vi "Weather Parse Test.vi"() -> ()   [LabVIEW 2020, in "CDM-Config.lvlib"] (continued)
    \"UGC\": [\n                        \"PKZ662\"\n                    ]\n                },\n                \"affectedZones\": [\n                    \"https://api.weather.gov/zones/forecast/PKZ662\"\n                ],\n                \"references\": [],\n                \"sent\": \"2025-12-02T14:58:00-09:00\",\n                \"effective\": \"2025-12-02T14:58:00-09:00\",\n                \"onset\": \"2025-12-02T14:00:00-09:00\",\n                \"expires\": \"2025-12-03T09:00:00-09:00\",\n                \"ends\": \"2025-12-03T17:00:00-09:00\",\n                \"status\": \"Actual\",\n                \"messageType\": \"Alert\",\n                \"category\": \"Met\",\n                \"severity\": \"Minor\",\n                \"certainty\": \"Likely\",\n                \"urgency\": \"Expected\",\n                \"event\": \"Small Craft Advisory\",\n                \"sender\": \"w-nws.webmaster@noaa.gov\",\n                \"senderName\": \"NWS Juneau AK\",\n                \"headline\": \"Small Craft Advisory issued December 2 at 2:58PM AKST until December 3 at 5:00PM AKST by NWS Juneau AK\",\n                \"description\": \"Southeast Alaska Coastal Waters from Dixon Entrance to\\nCape Suckling out 100 NM\\n\\nWind forecasts reflect the predominant speed and direction\\nexpected. Seas forecasts represent the average of the highest\\none-third of the combined windwave and swell height.\\n\\n.TONIGHT...S wind 25 kt. Seas 11 ft. Rain.\\n.WED...SW wind 15 kt. Seas 11 ft. SW swell.\\n.WED NIGHT...W wind 20 kt. Seas 10 ft.\\n.THU...W wind 10 kt. Seas 9 ft.\\n.THU NIGHT...SE wind 20 kt. Seas 9 ft.\\n.FRI...W wind 25 kt. Seas 14 ft.\\n.SAT...S wind 30 kt. Seas 17 ft.\\n.SUN...SW gale to 35 kt. Seas 20 ft.\",\n                \"instruction\": null,\n                \"response\": \"Avoid\",\n                \"parameters\": {\n                    \"AWIPSidentifier\": [\n                        \"CWFAEG\"\n                    ],\n                    \"WMOidentifier\": [\n                        \"FZAK52 PAJK 022358\"\n                    ],\n                    \"NWSheadline\": [\n                        \"SMALL CRAFT ADVISORY THROUGH WEDNESDAY\"\n                    ],\n                    \"BLOCKCHANNEL\": [\n                        \"EAS\",\n                        \"NWEM\",\n                        \"CMAS\"\n                    ],\n                    \"VTEC\": [\n                        \"/O.NEW.PAJK.SC.Y.1226.251202T2300Z-251204T0200Z/\"\n                    ],\n                    \"eventEndingTime\": [\n                        \"2025-12-03T17:00:00-09:00\"\n                    ]\n                },\n                \"scope\": \"Public\",\n                \"code\": \"IPAWSv1.0\",\n                \"language\": \"en-US\",\n                \"web\": \"http://www.weather.gov\",\n                \"eventCode\": {\n                    \"SAME\": [\n                        \"NWS\"\n                    ],\n                    \"NationalWeatherService\": [\n                        \"SCY\"\n                    ]\n                }\n            }\n        },\n        {\n            \"id\": \"https://api.weather.gov/alerts/urn:oid:2.49.0.1.840.0.63d5e98d8e0beb997c67cb867ab3ed73fdae0812.009.1\",\n            \"type\": \"Feature\",\n            \"geometry\": null,\n            \"properties\": {\n                \"@id\": \"https://api.weather.gov/alerts/urn:oid:2.49.0.1.840.0.63d5e98d8e0beb997c67cb867ab3ed73fdae0812.009.1\",\n                \"@type\": \"wx:Alert\",\n                \"id\": \"urn:oid:2.49.0.1.840.0.63d5e98d8e0beb997c67cb867ab3ed73fdae0812.009.1\",\n                \"areaDesc\": \"Cape Spencer to Cape Fairweather from 15 to 85 NM\",\n                \"geocode\": {\n                    \"SAME\": [\n                        \"058664\"\n                    ],\n                    \"UGC\": [\n                        \"PKZ664\"\n                    ]\n                },\n                \"affectedZones\": [\n                    \"https://api.weather.gov/zones/forecast/PKZ664\"\n                ],\n                \"references\": [],\n                \"sent\": \"2025-12-02T14:58:00-09:00\",\n                \"effective\": \"2025-12-02T14:58:00-09:00\",\n                \"onset\": \"2025-12-02T14:00:00-09:00\",\n                \"expires\": \"2025-12-03T09:00:00-09:00\",\n                \"ends\": \"2025-12-03T17:00:00-09:00\",\n                \"status\": \"Actual\",\n                \"messageType\": \"Alert\",\n                \"category\": \"Met\",\n                \"severity\": \"Minor\",\n                \"certainty\": \"Likely\",\n                \"urgency\": \"Expected\",\n                \"event\": \"Small Craft Advisory\",\n                \"sender\": \"w-nws.webmaster@noaa.gov\",\n                \"senderName\": \"NWS Juneau AK\",\n                \"headline\": \"Small Craft Advisory issued December 2 at 2:58PM AKST until December 3 at 5:00PM AKST by NWS Juneau AK\",\n                \"description\": \"Southeast Alaska Coastal Waters from Dixon Entrance to\\nCape Suckling out 100 NM\\n\\nWind forecasts reflect the predominant speed and direction\\nexpected. Seas forecasts represent the average of the highest\\none-third of the combined windwave and swell height.\\n\\n.TONIGHT...SE wind 20 kt. Seas 11 ft. Rain in the evening.\\n.WED...S wind 20 kt becoming W in the afternoon. Seas\\n12 ft. SW swell.\\n.WED NIGHT...W wind 20 kt. Seas 10 ft.\\n.THU...W wind 15 kt. Seas 9 ft.\\n.THU NIGHT...SE wind 20 kt. Seas 8 ft.\\n.FRI...SW wind 25 kt. Seas 9 ft.\\n.SAT...S gale to 35 kt. Seas 14 ft.\\n.SUN...S gale to 35 kt. Seas 18 ft.\",\n                \"instruction\": null,\n                \"response\": \"Avoid\",\n                \"parameters\": {\n                    \"AWIPSidentifier\": [\n                        \"CWFAEG\"\n                    ],\n                    \"WMOidentifier\": [\n                        \"FZAK52 PAJK 022358\"\n                    ],\n                    \"NWSheadline\": [\n                        \"SMALL CRAFT ADVISORY THROUGH WEDNESDAY\"\n                    ],\n                    \"BLOCKCHANNEL\": [\n                        \"EAS\",\n                        \"NWEM\",\n                        \"CMAS\"\n                    ],\n                    \"VTEC\": [\n                        \"/O.NEW.PAJK.SC.Y.1230.251202T2300Z-251204T0200Z/\"\n                    ],\n                    \"eventEndingTime\": [\n                        \"2025-12-03T17:00:00-09:00\"\n                    ]\n                },\n                \"scope\": \"Public\",\n                \"code\": \"IPAWSv1.0\",\n                \"language\": \"en-US\",\n                \"web\": \"http://www.weather.gov\",\n                \"eventCode\": {\n                    \"SAME\": [\n                        \"NWS\"\n                    ],\n                    \"NationalWeatherService\": [\n                        \"SCY\"\n                    ]\n                }\n            }\n        },\n        {\n            \"id\": \"https://api.weather.gov/alerts/urn:oid:2.49.0.1.840.0.63d5e98d8e0beb997c67cb867ab3ed73fdae0812.013.1\",\n            \"type\": \"Feature\",\n            \"geometry\": null,\n            \"properties\": {\n                \"@id\": \"https://api.weather.gov/alerts/urn:oid:2.49.0.1.840.0.63d5e98d8e0beb997c67cb867ab3ed73fdae0812.013.1\",\n                \"@type\": \"wx:Alert\",\n                \"id\": \"urn:oid:2.49.0.1.840.0.63d5e98d8e0beb997c67cb867ab3ed73fdae0812.013.1\",\n                \"areaDesc\": \"Icy Cape to Cape Suckling from 15 to 80 NM\",\n                \"geocode\": {\n                    \"SAME\": [\n                        \"058672\"\n                    ],\n                    \"UGC\": [\n                        \"PKZ672\"\n                    ]\n                },\n                \"affectedZones\": [\n                    \"https://api.weather.gov/zones/forecast/PKZ672\"\n                ],\n                \"references\": [],\n                \"sent\": \"2025-12-02T14:58:00-09:00\",\n                \"effective\": \"2025-12-02T14:58:00-09:00\",\n                \"onset\": \"2025-12-02T14:00:00-09:00\",\n                \"expires\": \"2025-12-03T09:00:00-09:00\",\n                \"ends\": \"2025-12-03T17:00:00-09:00\",\n                \"status\": \"Actual\",\n                \"messageType\": \"Alert\",\n                \"category\": \"Met\",\n                \"severity\": \"Minor\",\n                \"certainty\": \"Likely\",\n                \"urgency\": \"Expected\",\n                \"event\": \"Small Craft Advisory\",\n                \"sender\": \"w-nws.webmaster@noaa.gov\",\n                \"senderName\": \"NWS Juneau AK\",\n                \"headline\": \"Small Craft Advisory issued December 2 at 2:58PM AKST until December 3 at 5:00PM AKST by NWS Juneau AK\",\n                \"description\": \"Southeast Alaska Coastal Waters from Dixon Entrance to\\nCape Suckling out 100 NM\\n\\nWind forecasts reflect the predominant speed and direction\\nexpected. Seas forecasts represent the average of the highest\\none-third of the combined windwave and swell height.\\n\\n.TONIGHT...E wind 25 kt. Seas 12 ft. Rain early in the evening.\\n.WED...E wind 20 kt becoming W in the afternoon. Seas\\n12 ft.\\n.WED NIGHT...W wind 15 kt. Seas 10 ft.\\n.THU...SW wind 10 kt. Seas 8 ft. SW swell.\\n.THU NIGHT...E wind 10 kt. Seas 8 ft.\\n.FRI...S wind 20 kt. Seas 8 ft.\\n.SAT...SE wind 30 kt. Seas 13 ft.\\n.SUN...SE gale to 35 kt. Seas 15 ft.\",\n                \"instruction\": null,\n                \"response\": \"Avoid\",\n                \"parameters\": {\n                    \"AWIPSidentifier\": [\n                        \"CWFAEG\"\n                    ],\n                    \"WMOidentifier\": [\n                        \"FZAK52 PAJK 022358\"\n                    ],\n                    \"NWSheadline\": [\n                        \"SMALL CRAFT ADVISORY THROUGH WEDNESDAY\"\n                    ],\n                    \"BLOCKCHANNEL\": [\n                        \"EAS\",\n                        \"NWEM\",\n                        \"CMAS\"\n                    ],\n                    \"VTEC\": [\n                        \"/O.NEW.PAJK.SC.Y.1234.251202T2300Z-251204T0200Z/\"\n                    ],\n                    \"eventEndingTime\": [\n                        \"2025-12-03T17:00:00-09:00\"\n                    ]\n                },\n                \"scope\": \"Public\",\n                \"code\": \"IPAWSv1.0\",\n                \"language\": \"en-US\",\n                \"web\": \"http://www.weather.gov\",\n                \"eventCode\": {\n                    \"SAME\": [\n                        \"NWS\"\n                    ],\n                    \"NationalWeatherService\": [\n                        \"SCY\"\n                    ]\n                }\n            }\n        },\n        {\n            \"id\": \"https://api.weather.gov/alerts/urn:oid:2.49.0.1.840.0.63d5e98d8e0beb997c67cb867ab3ed73fdae0812.002.1\",\n            \"type\": \"Feature\",\n            \"geometry\": null,\n            \"properties\": {\n                \"@id\": \"https://api.weather.gov/alerts/urn:oid:2.49.0.1.840.0.63d5e98d8e0beb997c67cb867ab3ed73fdae0812.002.1\",\n                \"@type\": \"wx:Alert\",\n                \"id\": \"urn:oid:2.49.0.1.840.0.63d5e98d8e0beb997c67cb867ab3ed73fdae0812.002.1\",\n                \"areaDesc\": \"Dixon Entrance to Cape Decision out to 15 NM\",\n                \"geocode\": {\n                    \"SAME\": [\n                        \"058641\"\n                    ],\n                    \"UGC\": [\n                        \"PKZ641\"\n                    ]\n                },\n                \"affectedZones\": [\n                    \"https://api.weather.gov/zones/forecast/PKZ641\"\n                ],\n                \"references\": [],\n                \"sent\": \"2025-12-02T14:58:00-09:00\",\n                \"effective\": \"2025-12-02T14:58:00-09:00\",\n                \"onset\": \"2025-12-02T14:00:00-09:00\",\n                \"expires\": \"2025-12-03T09:00:00-09:00\",\n                \"ends\": \"2025-12-03T17:00:00-09:00\",\n                \"status\": \"Actual\",\n                \"messageType\": \"Alert\",\n                \"category\": \"Met\",\n                \"severity\": \"Minor\",\n                \"certainty\": \"Likely\",\n                \"urgency\": \"Expected\",\n                \"event\": \"Small Craft Advisory\",\n                \"sender\": \"w-nws.webmaster@noaa.gov\",\n                \"senderName\": \"NWS Juneau AK\",\n                \"headline\": \"Small Craft Advisory issued December 2 at 2:58PM AKST until December 3 at 5:00PM AKST by NWS Juneau AK\",\n                \"description\": \"Southeast Alaska Coastal Waters from Dixon Entrance to\\nCape Suckling out 100 NM\\n\\nWind forecasts reflect the predominant speed and direction\\nexpected. Seas forecasts represent the average of the highest\\none-third of the combined windwave and swell height.\\n\\n.TONIGHT...SE wind 20 kt. Seas 11 ft. Rain.\\n.WED...S wind 20 kt becoming W in the afternoon. Seas\\n11 ft. Rain in the morning.\\n.WED NIGHT...W wind 15 kt. Seas 10 ft.\\n.THU...W wind 10 kt. Seas 8 ft. SW swell.\\n.THU NIGHT...SE wind 20 kt. Seas 9 ft. Rain.\\n.FRI...W wind 25 kt. Seas 15 ft.\\n.SAT...S wind 30 kt. Seas 15 ft.\\n.SUN...S gale to 35 kt. Seas 18 ft.\",\n                \"instruction\": null,\n                \"response\": \"Avoid\",\n                \"parameters\": {\n                    \"AWIPSidentifier\": [\n                        \"CWFAEG\"\n                    ],\n                    \"WMOidentifier\": [\n                        \"FZAK52 PAJK 022358\"\n                    ],\n                    \"NWSheadline\": [\n                        \"SMALL CRAFT ADVISORY THROUGH WEDNESDAY\"\n                    ],\n                    \"BLOCKCHANNEL\": [\n                        \"EAS\",\n                        \"NWEM\",\n                        \"CMAS\"\n                    ],\n                    \"VTEC\": [\n                        \"/O.NEW.PAJK.SC.Y.1223.251202T2300Z-251204T0200Z/\"\n                    ],\n                    \"eventEndingTime\": [\n                        \"2025-12-03T17:00:00-09:00\"\n                    ]\n                },\n                \"scope\": \"Public\",\n                \"code\": \"IPAWSv1.0\",\n                \"language\": \"en-US\",\n                \"web\": \"http://www.weather.gov\",\n                \"eventCode\": {\n                    \"SAME\": [\n                        \"NWS\"\n                    ],\n                    \"NationalWeatherService\": [\n                        \"SCY\"\n                    ]\n                }\n            }\n        },\n        {\n            \"id\": \"https://api.weather.gov/alerts/urn:oid:2.49.0.1.840.0.63d5e98d8e0beb997c67cb867ab3ed73fdae0812.004.1\",\n            \"type\": \"Feature\",\n            \"geometry\": null,\n            \"properties\": {\n                \"@id\": \"https://api.weather.gov/alerts/urn:oid:2.49.0.1.840.0.63d5e98d8e0beb997c67cb867ab3ed73fdae0812.004.1\",\n                \"@type\": \"wx:Alert\",\n                \"id\": \"urn:oid:2.49.0.1.840.0.63d5e98d8e0beb997c67cb867ab3ed73fdae0812.004.1\",\n                \"areaDesc\": \"Cape Decision to Cape Edgecumbe out to 15 NM\",\n                \"geocode\": {\n                    \"SAME\": [\n                        \"058642\"\n                    ],\n                    \"UGC\": [\n                        \"PKZ642\"\n                    ]\n                },\n                \"affectedZones\": [\n                    \"https://api.weather.gov/zones/forecast/PKZ642\"\n                ],\n                \"references\": [],\n                \"sent\": \"2025-12-02T14:58:00-09:00\",\n                \"effective\": \"2025-12-02T14:58:00-09:00\",\n                \"onset\": \"2025-12-02T14:00:00-09:00\",\n                \"expires\": \"2025-12-03T09:00:00-09:00\",\n                \"ends\": \"2025-12-03T17:00:00-09:00\",\n                \"status\": \"Actual\",\n                \"messageType\": \"Alert\",\n                \"category\": \"Met\",\n                \"severity\": \"Minor\",\n                \"certainty\": \"Likely\",\n                \"urgency\": \"Expected\",\n                \"event\": \"Small Craft Advisory\",\n                \"sender\": \"w-nws.webmaster@noaa.gov\",\n                \"senderName\": \"NWS Juneau AK\",\n                \"headline\": \"Small Craft Advisory issued December 2 at 2:58PM AKST until December 3 at 5:00PM AKST by NWS Juneau AK\",\n                \"description\": \"Southeast Alaska Coastal Waters from Dixon Entrance to\\nCape Suckling out 100 NM\\n\\nWind forecasts reflect the predominant speed and direction\\nexpected. Seas forecasts represent the average of the highest\\none-third of the combined windwave and swell height.\\n\\n.TONIGHT...S wind 15 kt becoming SE 25 kt. Seas 11 ft. Rain.\\n.WED...SW wind 15 kt. Seas 11 ft. Rain in the morning.\\n.WED NIGHT...W wind 15 kt. Seas 10 ft.\\n.THU...W wind 10 kt. Seas 9 ft.\\n.THU NIGHT...E wind 20 kt. Seas 9 ft.\\n.FRI...W wind 20 kt. Seas 13 ft.\\n.SAT...S wind 30 kt. Seas 16 ft.\\n.SUN...S gale to 35 kt. Seas 18 ft.\",\n                \"instruction\": null,\n                \"response\": \"Avoid\",\n                \"parameters\": {\n                    \"AWIPSidentifier\": [\n                        \"CWFAEG\"\n                    ],\n                    \"WMOidentifier\": [\n                        \"FZAK52 PAJK 022358\"\n                    ],\n                    \"NWSheadline\": [\n                        \"SMALL CRAFT ADVISORY THROUGH WEDNESDAY\"\n                    ],\n                    \"BLOCKCHANNEL\": [\n                        \"EAS\",\n                        \"NWEM\",\n                        \"CMAS\"\n                    ],\n                    \"VTEC\": [\n                        \"/O.NEW.PAJK.SC.Y.1225.251202T2300Z-251204T0200Z/\"\n                    ],\n                    \"eventEndingTime\": [\n                        \"2025-12-03T17:00:00-09:00\"\n                    ]\n                },\n                \"scope\": \"Public\",\n                \"code\": \"IPAWSv1.0\",\n                \"language\": \"en-US\",\n                \"web\": \"http://www.weather.gov\",\n                \"eventCode\": {\n                    \"SAME\": [\n                        \"NWS\"\n                    ],\n                    \"NationalWeatherService\": [\n                        \"SCY\"\n                    ]\n                }\n            }\n        },\n        {\n            \"id\": \"https://api.weather.gov/alerts/urn:oid:2.49.0.1.840.0.63d5e98d8e0beb997c67cb867ab3ed73fdae0812.011.1\",\n            \"type\": \"Feature\",\n            \"geometry\": null,\n            \"properties\": {\n                \"@id\": \"https://api.weather.gov/alerts/urn:oid:2.49.0.1.840.0.63d5e98d8e0beb997c67cb867ab3ed73fdae0812.011.1\",\n                \"@type\": \"wx:Alert\",\n                \"id\": \"urn:oid:2.49.0.1.840.0.63d5e98d8e0beb997c67cb867ab3ed73fdae0812.011.1\",\n                \"areaDesc\": \"Cape Fairweather to Icy Cape from 15 to 80 NM\",\n                \"geocode\": {\n                    \"SAME\": [\n                        \"058671\"\n                    ],\n                    \"UGC\": [\n                        \"PKZ671\"\n                    ]\n                },\n                \"affectedZones\": [\n                    \"https://api.weather.gov/zones/forecast/PKZ671\"\n                ],\n                \"references\": [],\n                \"sent\": \"2025-12-02T14:58:00-09:00\",\n                \"effective\": \"2025-12-02T14:58:00-09:00\",\n                \"onset\": \"2025-12-02T14:00:00-09:00\",\n                \"expires\": \"2025-12-03T09:00:00-09:00\",\n                \"ends\": \"2025-12-03T17:00:00-09:00\",\n                \"status\": \"Actual\",\n                \"messageType\": \"Alert\",\n                \"category\": \"Met\",\n                \"severity\": \"Minor\",\n                \"certainty\": \"Likely\",\n                \"urgency\": \"Expected\",\n                \"event\": \"Small Craft Advisory\",\n                \"sender\": \"w-nws.webmaster@noaa.gov\",\n                \"senderName\": \"NWS Juneau AK\",\n                \"headline\": \"Small Craft Advisory issued December 2 at 2:58PM AKST until December 3 at 5:00PM AKST by NWS Juneau AK\",\n                \"description\": \"Southeast Alaska Coastal Waters from Dixon Entrance to\\nCape Suckling out 100 NM\\n\\nWind forecasts reflect the predominant speed and direction\\nexpected. Seas forecasts represent the average of the highest\\none-third of the combined windwave and swell height.\\n\\n.TONIGHT...SE wind 25 kt. Seas 11 ft. Rain in the evening.\\n.WED...S wind 25 kt becoming SW 15 kt in the afternoon.\\nSeas 12 ft. SW swell. Rain in the morning.\\n.WED NIGHT...W wind 20 kt. Seas 10 ft.\\n.THU...W wind 10 kt. Seas 9 ft.\\n.THU NIGHT...E wind 15 kt. Seas 8 ft.\\n.FRI...S wind 25 kt. Seas 9 ft.\\n.SAT...SE wind 30 kt. Seas 14 ft.\\n.SUN...SE gale to 35 kt. Seas 16 ft.\",\n                \"instruction\": null,\n                \"response\": \"Avoid\",\n                \"parameters\": {\n                    \"AWIPSidentifier\": [\n                        \"CWFAEG\"\n                    ],\n                    \"WMOidentifier\": [\n                        \"FZAK52 PAJK 022358\"\n                    ],\n                    \"NWSheadline\": [\n                        \"SMALL CRAFT ADVISORY THROUGH WEDNESDAY\"\n                    ],\n                    \"BLOCKCHANNEL\": [\n                        \"EAS\",\n                        \"NWEM\",\n                        \"CMAS\"\n                    ],\n                    \"VTEC\": [\n                        \"/O.NEW.PAJK.SC.Y.1232.251202T2300Z-251204T0200Z/\"\n                    ],\n                    \"eventEndingTime\": [\n                        \"2025-12-03T17:00:00-09:00\"\n                    ]\n                },\n                \"scope\": \"Public\",\n                \"code\": \"IPAWSv1.0\",\n                \"language\": \"en-US\",\n                \"web\": \"http://www.weather.gov\",\n                \"eventCode\": {\n                    \"SAME\": [\n                        \"NWS\"\n                    ],\n                    \"NationalWeatherService\": [\n                        \"SCY\"\n                    ]\n                }\n            }\n        },\n        {\n            \"id\": \"https://api.weather.gov/alerts/urn:oid:2.49.0.1.840.0.cd90ac8a87561bc2b815ad8e2c96450855688a45.001.1\",\n            \"type\": \"Feature\",\n            \"geometry\": null,\n            \"properties\": {\n                \"@id\": \"https://api.weather.gov/alerts/urn:oid:2.49.0.1.840.0.cd90ac8a87561bc2b815ad8e2c96450855688a45.001.1\",\n                \"@type\": \"wx:Alert\",\n                \"id\": \"urn:oid:2.49.0.1.840.0.cd90ac8a87561bc2b815ad8e2c96450855688a45.001.1\",\n                \"areaDesc\": \"City and Borough of Yakutat; Municipality of Skagway; Haines Borough and Klukwan\",\n                \"geocode\": {\n                    \"SAME\": [\n                        \"002282\",\n                        \"002230\",\n                        \"002100\"\n                    ],\n                    \"UGC\": [\n                        \"AKZ317\",\n                        \"AKZ318\",\n                        \"AKZ319\"\n                    ]\n                },\n                \"affectedZones\": [\n                    \"https://api.weather.gov/zones/forecast/AKZ317\",\n                    \"https://api.weather.gov/zones/forecast/AKZ318\",\n                    \"https://api.weather.gov/zones/forecast/AKZ319\"\n                ],\n                \"references\": [],\n                \"sent\": \"2025-12-02T14:57:00-09:00\",\n                \"effective\": \"2025-12-02T14:57:00-09:00\",\n                \"onset\": \"2025-12-02T14:57:00-09:00\",\n                \"expires\": \"2025-12-03T15:00:00-09:00\",\n                \"ends\": null,\n                \"status\": \"Actual\",\n                \"messageType\": \"Alert\",\n                \"category\": \"Met\",\n                \"severity\": \"Moderate\",\n                \"certainty\": \"Observed\",\n                \"urgency\": \"Expected\",\n                \"event\": \"Special Weather Statement\",\n                \"sender\": \"w-nws.webmaster@noaa.gov\",\n                \"senderName\": \"NWS Juneau AK\",\n                \"headline\": \"Special Weather Statement issued December 2 at 2:57PM AKST by NWS Juneau AK\",\n                \"description\": \"Multiple systems look to move through the region this coming\\nweekend. Temperatures and snow levels are expected to steadily\\nfall starting Friday night across Yakutat and the Northern Inner\\nChannels.\\n\\nSnowfall rates will increase Saturday with potential for 6 inches\\nevery 12 hours and at least a 20% probability of 24 hour\\naccumulations exceeding 12 inches.\\n\\nSnow is likely to continue through Sunday and potentially into\\nMonday as additional weather systems move into the region. Stay\\ntuned to the forecast over the coming days. Now is the time to\\nbegin preparations for this potentially significant event.\",\n                \"instruction\": null,\n                \"response\": \"Execute\",\n                \"parameters\": {\n                    \"AWIPSidentifier\": [\n                        \"SPSAJK\"\n                    ],\n                    \"WMOidentifier\": [\n                        \"WWAK87 PAJK 022357\"\n                    ],\n                    \"NWSheadline\": [\n                        \"POTENTIAL FOR SIGNIFICANT LONG DURATION SNOW EVENT THIS WEEKEND\"\n                    ],\n                    \"BLOCKCHANNEL\": [\n                        \"EAS\",\n                        \"NWEM\",\n                        \"CMAS\"\n                    ],\n                    \"EAS-ORG\": [\n                        \"WXR\"\n                    ]\n                },\n                \"scope\": \"Public\",\n                \"code\": \"IPAWSv1.0\",\n                \"language\": \"en-US\",\n                \"web\": \"http://www.weather.gov\",\n                \"eventCode\": {\n                    \"SAME\": [\n                        \"SPS\"\n                    ],\n                    \"NationalWeatherService\": [\n                        \"SPS\"\n                    ]\n                }\n            }\n        },\n        {\n            \"id\": \"https://api.weather.gov/alerts/urn:oid:2.49.0.1.840.0.cd90ac8a87561bc2b815ad8e2c96450855688a45.002.1\",\n            \"type\": \"Feature\",\n            \"geometry\": null,\n            \"properties\": {\n                \"@id\": \"https://api.weather.gov/alerts/urn:oid:2.49.0.1.840.0.cd90ac8a87561bc2b815ad8e2c96450855688a45.002.1\",\n                \"@type\": \"wx:Alert\",\n                \"id\": \"urn:oid:2.49.0.1.840.0.cd90ac8a87561bc2b815ad8e2c96450855688a45.002.1\",\n                \"areaDesc\": \"Glacier Bay; Eastern Chichagof Island; Cape Fairweather to Lisianski Strait; City and Borough of Juneau\",\n                \"geocode\": {\n                    \"SAME\": [\n                        \"002105\",\n                        \"002110\"\n                    ],\n                    \"UGC\": [\n                        \"AKZ320\",\n                        \"AKZ321\",\n                        \"AKZ322\",\n                        \"AKZ325\"\n                    ]\n                },\n                \"affectedZones\": [\n                    \"https://api.weather.gov/zones/forecast/AKZ320\",\n                    \"https://api.weather.gov/zones/forecast/AKZ321\",\n                    \"https://api.weather.gov/zones/forecast/AKZ322\",\n                    \"https://api.weather.gov/zones/forecast/AKZ325\"\n                ],\n                \"references\": [],\n                \"sent\": \"2025-12-02T14:57:00-09:00\",\n                \"effective\": \"2025-12-02T14:57:00-09:00\",\n                \"onset\": \"2025-12-02T14:57:00-09:00\",\n                \"expires\": \"2025-12-03T15:00:00-09:00\",\n                \"ends\": null,\n                \"status\": \"Actual\",\n                \"messageType\": \"Alert\",\n                \"category\": \"Met\",\n                \"severity\": \"Moderate\",\n                \"certainty\": \"Observed\",\n                \"urgency\": \"Expected\",\n                \"event\": \"Special Weather Statement\",\n                \"sender\": \"w-nws.webmaster@noaa.gov\",\n                \"senderName\": \"NWS Juneau AK\",\n                \"headline\": \"Special Weather Statement issued December 2 at 2:57PM AKST by NWS Juneau AK\",\n                \"description\": \"..POTENTIAL FOR SIGNIFICANT LONG DURATION SNOW EVENT LATE THIS\\nWEEKEND...\\n\\nMultiple systems look to move through the region this coming\\nweekend. Temperatures and snow levels are expected to steadily\\nfall on Sunday over the Juneau and Icy Strait areas.\\n\\nSnowfall rates will increase through Sunday with potential for 6\\ninches every 12 hours and at least a 20% probability of 24 hour\\naccumulations exceeding 12 inches.\\n\\nSnow is likely to continue through Monday and potentially longer\\nas additional weather systems move into the region. Stay tuned to\\nthe forecast over the coming days. Now is the time to begin\\npreparations for this potentially significant event.\",\n                \"instruction\": null,\n                \"response\": \"Execute\",\n                \"parameters\": {\n                    \"AWIPSidentifier\": [\n                        \"SPSAJK\"\n                    ],\n                    \"WMOidentifier\": [\n                        \"WWAK87 PAJK 022357\"\n                    ],\n                    \"BLOCKCHANNEL\": [\n                        \"EAS\",\n                        \"NWEM\",\n                        \"CMAS\"\n                    ],\n                    \"EAS-ORG\": [\n                        \"WXR\"\n                    ]\n                },\n                \"scope\": \"Public\",\n                \"code\": \"IPAWSv1.0\",\n                \"language\": \"en-US\",\n                \"web\": \"http://www.weather.gov\",\n                \"eventCode\": {\n                    \"SAME\": [\n                        \"SPS\"\n                    ],\n                    \"NationalWeatherService\": [\n                        \"SPS\"\n                    ]\n                }\n            }\n        },\n        {\n            \"id\": \"https://api.weather.gov/alerts/urn:oid:2.49.0.1.840.0.ed8afaf6a4e163dc7575337e7e142512eec7886f.001.1\",\n            \"type\": \"Feature\",\n            \"geometry\": null,\n            \"properties\": {\n                \"@id\": \"https://api.weather.gov/alerts/urn:oid:2.49.0.1.840.0.ed8afaf6a4e163dc7575337e7e142512eec7886f.001.1\",\n                \"@type\": \"wx:Alert\",\n                \"id\": \"urn:oid:2.49.0.1.840.0.ed8afaf6a4e163dc7575337e7e142512eec7886f.001.1\",\n                \"areaDesc\": \"South Slopes Of The Eastern Brooks Range; South Slopes Of The Central Brooks Range; Upper Koyukuk Valley\",\n                \"geocode\": {\n                    \"SAME\": [\n                        \"002290\"\n                    ],\n                    \"UGC\": [\n                        \"AKZ811\",\n                        \"AKZ812\",\n                        \"AKZ831\"\n                    ]\n                },\n                \"affectedZones\": [\n                    \"https://api.weather.gov/zones/forecast/AKZ811\",\n                    \"https://api.weather.gov/zones/forecast/AKZ812\",\n                    \"https://api.weather.gov/zones/forecast/AKZ831\"\n                ],\n                \"references\": [],\n                \"sent\": \"2025-12-02T13:18:00-09:00\",\n                \"effective\": \"2025-12-02T13:18:00-09:00\",\n                \"onset\": \"2025-12-02T13:18:00-09:00\",\n                \"expires\": \"2025-12-03T09:00:00-09:00\",\n                \"ends\": null,\n                \"status\": \"Actual\",\n                \"messageType\": \"Alert\",\n                \"category\": \"Met\",\n                \"severity\": \"Moderate\",\n                \"certainty\": \"Observed\",\n                \"urgency\": \"Expected\",\n                \"event\": \"Special Weather Statement\",\n                \"sender\": \"w-nws.webmaster@noaa.gov\",\n                \"senderName\": \"NWS Fairbanks AK\",\n                \"headline\": \"Special Weather Statement issued December 2 at 1:18PM AKST by NWS Fairbanks AK\",\n                \"description\": \"As of 1pm AKST Tuesday, 2 to 4 inches of snow have been reported\\nso far across the area. An additional 1 to 3 inches are expected\\nsoutheast of Bettles to Hughes and north of the White Mountains,\\nwhere more snow is expected. Snow will continue through Wednesday\\nmorning before tapering off.\",\n                \"instruction\": null,\n                \"response\": \"Execute\",\n                \"parameters\": {\n                    \"AWIPSidentifier\": [\n                        \"SPSAFG\"\n                    ],\n                    \"WMOidentifier\": [\n                        \"WWAK83 PAFG 022218\"\n                    ],\n                    \"NWSheadline\": [\n                        \"Moderate Snow Continues\"\n                    ],\n                    \"BLOCKCHANNEL\": [\n                        \"EAS\",\n                        \"NWEM\",\n                        \"CMAS\"\n                    ],\n                    \"EAS-ORG\": [\n                        \"WXR\"\n                    ]\n                },\n                \"scope\": \"Public\",\n                \"code\": \"IPAWSv1.0\",\n                \"language\": \"en-US\",\n                \"web\": \"http://www.weather.gov\",\n                \"eventCode\": {\n                    \"SAME\": [\n                        \"SPS\"\n                    ],\n                    \"NationalWeatherService\": [\n                        \"SPS\"\n                    ]\n                }\n            }\n        },\n        {\n            \"id\": \"https://api.weather.gov/alerts/urn:oid:2.49.0.1.840.0.7cc99ac4f72189d053b3bdd08312f3ca0c75fe30.024.1\",\n            \"type\": \"Feature\",\n            \"geometry\": null,\n            \"properties\": {\n                \"@id\": \"https://api.weather.gov/alerts/urn:oid:2.49.0.1.840.0.7cc99ac4f72189d053b3bdd08312f3ca0c75fe30.024.1\",\n                \"@type\": \"wx:Alert\",\n                \"id\": \"urn:oid:2.49.0.1.840.0.7cc99ac4f72189d053b3bdd08312f3ca0c75fe30.024.1\",\n                \"areaDesc\": \"Seguam to Adak Pacific Side from 15 to 75 NM\",\n                \"geocode\": {\n                    \"SAME\": [\n                        \"058783\"\n                    ],\n                    \"UGC\": [\n                        \"PKZ783\"\n                    ]\n                },\n                \"affectedZones\": [\n                    \"https://api.weather.gov/zones/forecast/PKZ783\"\n                ],\n                \"references\": [],\n                \"sent\": \"2025-12-02T07:08:00-09:00\",\n                \"effective\": \"2025-12-02T07:08:00-09:00\",\n                \"onset\": \"2025-12-02T07:00:00-09:00\",\n                \"expires\": \"2025-12-02T20:15:00-09:00\",\n                \"ends\": \"2025-12-03T17:00:00-09:00\",\n                \"status\": \"Actual\",\n                \"messageType\": \"Alert\",\n                \"category\": \"Met\",\n                \"severity\": \"Moderate\",\n                \"certainty\": \"Likely\",\n                \"urgency\": \"Expected\",\n                \"event\": \"Gale Warning\",\n                \"sender\": \"w-nws.webmaster@noaa.gov\",\n                \"senderName\": \"NWS Anchorage AK\",\n                \"headline\": \"Gale Warning issued December 2 at 7:08AM AKST until December 3 at 5:00PM AKST by NWS Anchorage AK\",\n                \"description\": \"Coastal Waters Forecast for Southwest Alaska+Bristol Bay+The\\nAlaska Peninsula Waters and the Aleutian Islands up to 100 nm out.\\n\\nWind forecasts reflect the predominant speed and direction\\nexpected. Sea forecasts represent an average of the highest\\none-third of the combined wind wave and swell height.\\n\\n.TODAY...N wind 45 kt. Seas 18 ft. Rain with snow.\\n.TONIGHT...NW wind 45 kt. Seas 20 ft.\\n.WED...N wind 35 kt. Seas 16 ft.\\n.WED NIGHT...N wind 30 kt. Seas 14 ft.\\n.THU...N wind 30 kt. Seas 11 ft.\\n.FRI...W wind 20 kt. Seas 15 ft.\\n.SAT...NE wind 15 kt. Seas 13 ft.\",\n                \"instruction\": null,\n                \"response\": \"Avoid\",\n                \"parameters\": {\n                    \"AWIPSidentifier\": [\n                        \"CWFALU\"\n                    ],\n                    \"WMOidentifier\": [\n                        \"FZAK52 PAFC 021608\"\n                    ],\n                    \"NWSheadline\": [\n                        \"GALE WARNING THROUGH WEDNESDAY\"\n                    ],\n                    \"BLOCKCHANNEL\": [\n                        \"EAS\",\n                        \"NWEM\",\n                        \"CMAS\"\n                    ],\n                    \"VTEC\": [\n                        \"/O.NEW.PAFC.GL.W.9091.251202T1600Z-251204T0200Z/\"\n                    ],\n                    \"eventEndingTime\": [\n                        \"2025-12-03T17:00:00-09:00\"\n                    ]\n                },\n                \"scope\": \"Public\",\n                \"code\": \"IPAWSv1.0\",\n                \"language\": \"en-US\",\n                \"web\": \"http://www.weather.gov\",\n                \"eventCode\": {\n                    \"SAME\": [\n                        \"NWS\"\n                    ],\n                    \"NationalWeatherService\": [\n                        \"GLW\"\n                    ]\n                }\n            }\n        },\n        {\n            \"id\": \"https://api.weather.gov/alerts/urn:oid:2.49.0.1.840.0.7cc99ac4f72189d053b3bdd08312f3ca0c75fe30.026.1\",\n            \"type\": \"Feature\",\n            \"geometry\": null,\n            \"properties\": {\n                \"@id\": \"https://api.weather.gov/alerts/urn:oid:2.49.0.1.840.0.7cc99ac4f72189d053b3bdd08312f3ca0c75fe30.026.1\",\n                \"@type\": \"wx:Alert\",\n                \"id\": \"urn:oid:2.49.0.1.840.0.7cc99ac4f72189d053b3bdd08312f3ca0c75fe30.026.1\",\n                \"areaDesc\": \"Adak to Kiska Pacific Side\",\n                \"geocode\": {\n                    \"SAME\": [\n                        \"058785\"\n                    ],\n                    \"UGC\": [\n                        \"PKZ785\"\n                    ]\n                },\n                \"affectedZones\": [\n                    \"https://api.weather.gov/zones/forecast/PKZ785\"\n                ],\n                \"references\": [],\n                \"sent\": \"2025-12-02T07:08:00-09:00\",\n                \"effective\": \"2025-12-02T07:08:00-09:00\",\n                \"onset\": \"2025-12-02T07:00:00-09:00\",\n                \"expires\": \"2025-12-02T20:15:00-09:00\",\n                \"ends\": \"2025-12-03T17:00:00-09:00\",\n                \"status\": \"Actual\",\n                \"messageType\": \"Alert\",\n                \"category\": \"Met\",\n                \"severity\": \"Moderate\",\n                \"certainty\": \"Likely\",\n                \"urgency\": \"Expected\",\n                \"event\": \"Gale Warning\",\n                \"sender\": \"w-nws.webmaster@noaa.gov\",\n                \"senderName\": \"NWS Anchorage AK\",\n                \"headline\": \"Gale Warning issued December 2 at 7:08AM AKST until December 3 at 5:00PM AKST by NWS Anchorage AK\",\n                \"description\": \"Coastal Waters Forecast for Southwest Alaska+Bristol Bay+The\\nAlaska Peninsula Waters and the Aleutian Islands up to 100 nm out.\\n\\nWind forecasts reflect the predominant speed and direction\\nexpected. Sea forecasts represent an average of the highest\\none-third of the combined wind wave and swell height.\\n\\n.TODAY...N wind 45 kt. Seas 24 ft.\\n.TONIGHT...N wind 40 kt. Seas 21 ft.\\n.WED...N wind 35 kt. Seas 20 ft.\\n.WED NIGHT...N wind 30 kt. Seas 15 ft.\\n.THU...E wind 30 kt. Seas 10 ft.\\n.FRI...W wind 25 kt. Seas 16 ft.\\n.SAT...E wind 15 kt. Seas 15 ft.\",\n                \"instruction\": null,\n                \"response\": \"Avoid\",\n                \"parameters\": {\n                    \"AWIPSidentifier\": [\n                        \"CWFALU\"\n                    ],\n                    \"WMOidentifier\": [\n                        \"FZAK52 PAFC 021608\"\n                    ],\n                    \"NWSheadline\": [\n                        \"GALE WARNING THROUGH WEDNESDAY\"\n                    ],\n                    \"BLOCKCHANNEL\": [\n                        \"EAS\",\n                        \"NWEM\",\n                        \"CMAS\"\n                    ],\n                    \"VTEC\": [\n                        \"/O.NEW.PAFC.GL.W.9093.251202T1600Z-251204T0200Z/\"\n                    ],\n                    \"eventEndingTime\": [\n                        \"2025-12-03T17:00:00-09:00\"\n                    ]\n                },\n                \"scope\": \"Public\",\n                \"code\": \"IPAWSv1.0\",\n                \"language\": \"en-US\",\n                \"web\": \"http://www.weather.gov\",\n                \"eventCode\": {\n                    \"SAME\": [\n                        \"NWS\"\n                    ],\n                    \"NationalWeatherService\": [\n                        \"GLW\"\n                    ]\n                }\n            }\n        },\n        {\n            \"id\": \"https://api.weather.gov/alerts/urn:oid:2.49.0.1.840.0.7cc99ac4f72189d053b3bdd08312f3ca0c75fe30.023.1\",\n            \"type\": \"Feature\",\n            \"geometry\": null,\n            \"properties\": {\n                \"@id\": \"https://api.weather.gov/alerts/urn:oid:2.49.0.1.840.0.7cc99ac4f72189d053b3bdd08312f3ca0c75fe30.023.1\",\n                \"@type\": \"wx:Alert\",\n                \"id\": \"urn:oid:2.49.0.1.840.0.7cc99ac4f72189d053b3bdd08312f3ca0c75fe30.023.1\",\n                \"areaDesc\": \"Seguam to Adak Pacific Side out to 15 NM\",\n                \"geocode\": {\n                    \"SAME\": [\n                        \"058782\"\n                    ],\n                    \"UGC\": [\n                        \"PKZ782\"\n                    ]\n                },\n                \"affectedZones\": [\n                    \"https://api.weather.gov/zones/forecast/PKZ782\"\n                ],\n                \"references\": [],\n                \"sent\": \"2025-12-02T07:08:00-09:00\",\n                \"effective\": \"2025-12-02T07:08:00-09:00\",\n                \"onset\": \"2025-12-02T07:00:00-09:00\",\n                \"expires\": \"2025-12-02T20:15:00-09:00\",\n                \"ends\": \"2025-12-03T17:00:00-09:00\",\n                \"status\": \"Actual\",\n                \"messageType\": \"Alert\",\n                \"category\": \"Met\",\n                \"severity\": \"Moderate\",\n                \"certainty\": \"Likely\",\n                \"urgency\": \"Expected\",\n                \"event\": \"Gale Warning\",\n                \"sender\": \"w-nws.webmaster@noaa.gov\",\n                \"senderName\": \"NWS Anchorage AK\",\n                \"headline\": \"Gale Warning issued December 2 at 7:08AM AKST until December 3 at 5:00PM AKST by NWS Anchorage AK\",\n                \"description\": \"Coastal Waters Forecast for Southwest Alaska+Bristol Bay+The\\nAlaska Peninsula Waters and the Aleutian Islands up to 100 nm out.\\n\\nWind forecasts reflect the predominant speed and direction\\nexpected. Sea forecasts represent an average of the highest\\none-third of the combined wind wave and swell height.\\n\\n.TODAY...N wind 45 kt. Seas 15 ft. Rain and snow.\\n.TONIGHT...N wind 45 kt. Seas 15 ft. Rain and snow.\\n.WED...N wind 35 kt. Seas 14 ft.\\n.WED NIGHT...N wind 30 kt. Seas 12 ft.\\n.THU...N wind 30 kt. Seas 9 ft.\\n.FRI...NW wind 15 kt. Seas 12 ft.\\n.SAT...NE wind 15 kt. Seas 12 ft.\",\n                \"instruction\": null,\n                \"response\": \"Avoid\",\n                \"parameters\": {\n                    \"AWIPSidentifier\": [\n                        \"CWFALU\"\n                    ],\n                    \"WMOidentifier\": [\n                        \"FZAK52 PAFC 021608\"\n                    ],\n                    \"NWSheadline\": [\n                        \"GALE WARNING THROUGH WEDNESDAY\"\n                    ],\n                    \"BLOCKCHANNEL\": [\n                        \"EAS\",\n                        \"NWEM\",\n                        \"CMAS\"\n                    ],\n                    \"VTEC\": [\n                        \"/O.NEW.PAFC.GL.W.9090.251202T1600Z-251204T0200Z/\"\n                    ],\n                    \"eventEndingTime\": [\n                        \"2025-12-03T17:00:00-09:00\"\n                    ]\n                },\n                \"scope\": \"Public\",\n                \"code\": \"IPAWSv1.0\",\n                \"language\": \"en-US\",\n                \"web\": \"http://www.weather.gov\",\n                \"eventCode\": {\n                    \"SAME\": [\n                        \"NWS\"\n                    ],\n                    \"NationalWeatherService\": [\n                        \"GLW\"\n                    ]\n                }\n            }\n        },\n        {\n            \"id\": \"https://api.weather.gov/alerts/urn:oid:2.49.0.1.840.0.7a1ebf60c096e67f68143934abaf6f7cf8a57038.005.1\",\n            \"type\": \"Feature\",\n            \"geometry\": null,\n            \"properties\": {\n                \"@id\": \"https://api.weather.gov/alerts/urn:oid:2.49.0.1.840.0.7a1ebf60c096e67f68143934abaf6f7cf8a57038.005.1\",\n                \"@type\": \"wx:Alert\",\n                \"id\": \"urn:oid:2.49.0.1.840.0.7a1ebf60c096e67f68143934abaf6f7cf8a57038.005.1\",\n                \"areaDesc\": \"Cape Cleare to Gore Point out to 15 NM\",\n                \"geocode\": {\n                    \"SAME\": [\n                        \"058715\"\n                    ],\n                    \"UGC\": [\n                        \"PKZ715\"\n                    ]\n                },\n                \"affectedZones\": [\n                    \"https://api.weather.gov/zones/forecast/PKZ715\"\n                ],\n                \"references\": [],\n                \"sent\": \"2025-12-02T02:49:00-09:00\",\n                \"effective\": \"2025-12-02T02:49:00-09:00\",\n                \"onset\": \"2025-12-02T02:00:00-09:00\",\n                \"expires\": \"2025-12-02T15:45:00-09:00\",\n                \"ends\": \"2025-12-03T17:00:00-09:00\",\n                \"status\": \"Actual\",\n                \"messageType\": \"Alert\",\n                \"category\": \"Met\",\n                \"severity\": \"Minor\",\n                \"certainty\": \"Likely\",\n                \"urgency\": \"Expected\",\n                \"event\": \"Small Craft Advisory\",\n                \"sender\": \"w-nws.webmaster@noaa.gov\",\n                \"senderName\": \"NWS Anchorage AK\",\n                \"headline\": \"Small Craft Advisory issued December 2 at 2:49AM AKST until December 3 at 5:00PM AKST by NWS Anchorage AK\",\n                \"description\": \"Coastal Waters Forecast for the Northern Gulf of Alaska Coast\\nup to 100 nm out including Kodiak Island and Cook Inlet.\\n\\nWind forecasts reflect the predominant speed and direction\\nexpected. Sea forecasts represent an average of the highest\\none-third of the combined wind wave and swell height.\\n\\n.TODAY...E wind 20 kt. Seas 8 ft. Rain.\\n.TONIGHT...Variable wind 10 kt. Seas 8 ft.\\n.WED...N wind 15 kt. Seas 8 ft.\\n.WED NIGHT...Variable wind 10 kt. Seas 8 ft.\\n.THU THROUGH FRI...Variable wind 10 kt. Seas 6 ft.\\n.SAT...NE wind 15 kt. Seas 7 ft.\",\n                \"instruction\": null,\n                \"response\": \"Avoid\",\n                \"parameters\": {\n                    \"AWIPSidentifier\": [\n                        \"CWFAER\"\n                    ],\n                    \"WMOidentifier\": [\n                        \"FZAK51 PAFC 021149\"\n                    ],\n                    \"NWSheadline\": [\n                        \"SMALL CRAFT ADVISORY THROUGH WEDNESDAY\"\n                    ],\n                    \"BLOCKCHANNEL\": [\n                        \"EAS\",\n                        \"NWEM\",\n                        \"CMAS\"\n                    ],\n                    \"VTEC\": [\n                        \"/O.NEW.PAFC.SC.Y.9560.251202T1100Z-251204T0200Z/\"\n                    ],\n                    \"eventEndingTime\": [\n                        \"2025-12-03T17:00:00-09:00\"\n                    ]\n                },\n                \"scope\": \"Public\",\n                \"code\": \"IPAWSv1.0\",\n                \"language\": \"en-US\",\n                \"web\": \"http://www.weather.gov\",\n                \"eventCode\": {\n                    \"SAME\": [\n                        \"NWS\"\n                    ],\n                    \"NationalWeatherService\": [\n                        \"SCY\"\n                    ]\n                }\n            }\n        },\n        {\n            \"id\": \"https://api.weather.gov/alerts/urn:oid:2.49.0.1.840.0.7a1ebf60c096e67f68143934abaf6f7cf8a57038.018.1\",\n            \"type\": \"Feature\",\n            \"geometry\": null,\n            \"properties\": {\n                \"@id\": \"https://api.weather.gov/alerts/urn:oid:2.49.0.1.840.0.7a1ebf60c096e67f68143934abaf6f7cf8a57038.018.1\",\n                \"@type\": \"wx:Alert\",\n                \"id\": \"urn:oid:2.49.0.1.840.0.7a1ebf60c096e67f68143934abaf6f7cf8a57038.018.1\",\n                \"areaDesc\": \"Marmot Island to Sitkinak out to 15 NM\",\n                \"geocode\": {\n                    \"SAME\": [\n                        \"058732\"\n                    ],\n                    \"UGC\": [\n                        \"PKZ732\"\n                    ]\n                },\n                \"affectedZones\": [\n                    \"https://api.weather.gov/zones/forecast/PKZ732\"\n                ],\n                \"references\": [],\n                \"sent\": \"2025-12-02T02:49:00-09:00\",\n                \"effective\": \"2025-12-02T02:49:00-09:00\",\n                \"onset\": \"2025-12-02T02:00:00-09:00\",\n                \"expires\": \"2025-12-02T15:45:00-09:00\",\n                \"ends\": \"2025-12-03T17:00:00-09:00\",\n                \"status\": \"Actual\",\n                \"messageType\": \"Alert\",\n                \"category\": \"Met\",\n                \"severity\": \"Minor\",\n                \"certainty\": \"Likely\",\n                \"urgency\": \"Expected\",\n                \"event\": \"Small Craft Advisory\",\n                \"sender\": \"w-nws.webmaster@noaa.gov\",\n                \"senderName\": \"NWS Anchorage AK\",\n                \"headline\": \"Small Craft Advisory issued December 2 at 2:49AM AKST until December 3 at 5:00PM AKST by NWS Anchorage AK\",\n                \"description\": \"Coastal Waters Forecast for the Northern Gulf of Alaska Coast\\nup to 100 nm out including Kodiak Island and Cook Inlet.\\n\\nWind forecasts reflect the predominant speed and direction\\nexpected. Sea forecasts represent an average of the highest\\none-third of the combined wind wave and swell height.\\n\\n.TODAY...S wind 30 kt diminishing to 15 kt in the afternoon. Seas\\n14 ft.\\n.TONIGHT...SE wind 20 kt. Seas 13 ft.\\n.WED...S wind 15 kt. Seas 11 ft.\\n.WED NIGHT...Variable wind 10 kt. Seas 9 ft.\\n.THU...NE wind 20 kt. Seas 8 ft.\\n.FRI...Variable wind 10 kt. Seas 6 ft.\\n.SAT...NW wind 20 kt. Seas 6 ft.\",\n                \"instruction\": null,\n                \"response\": \"Avoid\",\n                \"parameters\": {\n                    \"AWIPSidentifier\": [\n                        \"CWFAER\"\n                    ],\n                    \"WMOidentifier\": [\n                        \"FZAK51 PAFC 021149\"\n                    ],\n                    \"NWSheadline\": [\n                        \"SMALL CRAFT ADVISORY THROUGH WEDNESDAY\"\n                    ],\n                    \"BLOCKCHANNEL\": [\n                        \"EAS\",\n                        \"NWEM\",\n                        \"CMAS\"\n                    ],\n                    \"VTEC\": [\n                        \"/O.NEW.PAFC.SC.Y.9566.251202T1100Z-251204T0200Z/\"\n                    ],\n                    \"eventEndingTime\": [\n                        \"2025-12-03T17:00:00-09:00\"\n                    ]\n                },\n                \"scope\": \"Public\",\n                \"code\": \"IPAWSv1.0\",\n                \"language\": \"en-US\",\n                \"web\": \"http://www.weather.gov\",\n                \"eventCode\": {\n                    \"SAME\": [\n                        \"NWS\"\n                    ],\n                    \"NationalWeatherService\": [\n                        \"SCY\"\n                    ]\n                }\n            }\n        },\n        {\n            \"id\": \"https://api.weather.gov/alerts/urn:oid:2.49.0.1.840.0.7a1ebf60c096e67f68143934abaf6f7cf8a57038.006.1\",\n            \"type\": \"Feature\",\n            \"geometry\": null,\n            \"properties\": {\n                \"@id\": \"https://api.weather.gov/alerts/urn:oid:2.49.0.1.840.0.7a1ebf60c096e67f68143934abaf6f7cf8a57038.006.1\",\n                \"@type\": \"wx:Alert\",\n                \"id\": \"urn:oid:2.49.0.1.840.0.7a1ebf60c096e67f68143934abaf6f7cf8a57038.006.1\",\n                \"areaDesc\": \"Cape Cleare to Gore Point from 15 to 75 NM\",\n                \"geocode\": {\n                    \"SAME\": [\n                        \"058716\"\n                    ],\n                    \"UGC\": [\n                        \"PKZ716\"\n                    ]\n                },\n                \"affectedZones\": [\n                    \"https://api.weather.gov/zones/forecast/PKZ716\"\n                ],\n                \"references\": [],\n                \"sent\": \"2025-12-02T02:49:00-09:00\",\n                \"effective\": \"2025-12-02T02:49:00-09:00\",\n                \"onset\": \"2025-12-02T02:00:00-09:00\",\n                \"expires\": \"2025-12-02T15:45:00-09:00\",\n                \"ends\": \"2025-12-03T17:00:00-09:00\",\n                \"status\": \"Actual\",\n                \"messageType\": \"Alert\",\n                \"category\": \"Met\",\n                \"severity\": \"Minor\",\n                \"certainty\": \"Likely\",\n                \"urgency\": \"Expected\",\n                \"event\": \"Small Craft Advisory\",\n                \"sender\": \"w-nws.webmaster@noaa.gov\",\n                \"senderName\": \"NWS Anchorage AK\",\n                \"headline\": \"Small Craft Advisory issued December 2 at 2:49AM AKST until December 3 at 5:00PM AKST by NWS Anchorage AK\",\n                \"description\": \"Coastal Waters Forecast for the Northern Gulf of Alaska Coast\\nup to 100 nm out including Kodiak Island and Cook Inlet.\\n\\nWind forecasts reflect the predominant speed and direction\\nexpected. Sea forecasts represent an average of the highest\\none-third of the combined wind wave and swell height.\\n\\n.TODAY...SE wind 25 kt. Seas 10 ft.\\n.TONIGHT...Variable wind 10 kt. Seas 10 ft.\\n.WED...Variable wind 10 kt. Seas 10 ft.\\n.WED NIGHT...SW wind 15 kt. Seas 9 ft.\\n.THU...Variable wind 10 kt. Seas 8 ft.\\n.FRI...Variable wind 10 kt. Seas 6 ft.\\n.SAT...SE wind 15 kt. Seas 7 ft.\",\n                \"instruction\": null,\n                \"response\": \"Avoid\",\n                \"parameters\": {\n                    \"AWIPSidentifier\": [\n                        \"CWFAER\"\n                    ],\n                    \"WMOidentifier\": [\n                        \"FZAK51 PAFC 021149\"\n                    ],\n                    \"NWSheadline\": [\n                        \"SMALL CRAFT ADVISORY THROUGH WEDNESDAY\"\n                    ],\n                    \"BLOCKCHANNEL\": [\n                        \"EAS\",\n                        \"NWEM\",\n                        \"CMAS\"\n                    ],\n                    \"VTEC\": [\n                        \"/O.NEW.PAFC.SC.Y.9561.251202T1100Z-251204T0200Z/\"\n                    ],\n                    \"eventEndingTime\": [\n                        \"2025-12-03T17:00:00-09:00\"\n                    ]\n                },\n                \"scope\": \"Public\",\n                \"code\": \"IPAWSv1.0\",\n                \"language\": \"en-US\",\n                \"web\": \"http://www.weather.gov\",\n                \"eventCode\": {\n                    \"SAME\": [\n                        \"NWS\"\n                    ],\n                    \"NationalWeatherService\": [\n                        \"SCY\"\n                    ]\n                }\n            }\n        },\n        {\n            \"id\": \"https://api.weather.gov/alerts/urn:oid:2.49.0.1.840.0.7a1ebf60c096e67f68143934abaf6f7cf8a57038.002.1\",\n            \"type\": \"Feature\",\n            \"geometry\": null,\n            \"properties\": {\n                \"@id\": \"https://api.weather.gov/alerts/urn:oid:2.49.0.1.840.0.7a1ebf60c096e67f68143934abaf6f7cf8a57038.002.1\",\n                \"@type\": \"wx:Alert\",\n                \"id\": \"urn:oid:2.49.0.1.840.0.7a1ebf60c096e67f68143934abaf6f7cf8a57038.002.1\",\n                \"areaDesc\": \"Cape Suckling to Gravel Point out to 15 NM\",\n                \"geocode\": {\n                    \"SAME\": [\n                        \"058710\"\n                    ],\n                    \"UGC\": [\n                        \"PKZ710\"\n                    ]\n                },\n                \"affectedZones\": [\n                    \"https://api.weather.gov/zones/forecast/PKZ710\"\n                ],\n                \"references\": [],\n                \"sent\": \"2025-12-02T02:49:00-09:00\",\n                \"effective\": \"2025-12-02T02:49:00-09:00\",\n                \"onset\": \"2025-12-02T02:00:00-09:00\",\n                \"expires\": \"2025-12-02T15:45:00-09:00\",\n                \"ends\": \"2025-12-03T17:00:00-09:00\",\n                \"status\": \"Actual\",\n                \"messageType\": \"Alert\",\n                \"category\": \"Met\",\n                \"severity\": \"Minor\",\n                \"certainty\": \"Likely\",\n                \"urgency\": \"Expected\",\n                \"event\": \"Small Craft Advisory\",\n                \"sender\": \"w-nws.webmaster@noaa.gov\",\n                \"senderName\": \"NWS Anchorage AK\",\n                \"headline\": \"Small Craft Advisory issued December 2 at 2:49AM AKST until December 3 at 5:00PM AKST by NWS Anchorage AK\",\n                \"description\": \"Coastal Waters Forecast for the Northern Gulf of Alaska Coast\\nup to 100 nm out including Kodiak Island and Cook Inlet.\\n\\nWind forecasts reflect the predominant speed and direction\\nexpected. Sea forecasts represent an average of the highest\\none-third of the combined wind wave and swell height.\\n\\n.TODAY...E wind 25 kt. Seas 9 ft. Rain.\\n.TONIGHT...E wind 30 kt. Seas 10 ft. Rain.\\n.WED...E wind 20 kt. Seas 9 ft. Rain.\\n.WED NIGHT...Variable wind 10 kt. Seas 9 ft.\\n.THU...Variable wind 10 kt. Seas 7 ft.\\n.FRI...E wind 15 kt. Seas 6 ft.\\n.SAT...E wind 20 kt. Seas 9 ft.\",\n                \"instruction\": null,\n                \"response\": \"Avoid\",\n                \"parameters\": {\n                    \"AWIPSidentifier\": [\n                        \"CWFAER\"\n   
